vi "Periodic Tasks.vi"(8 "error in":errorcluster) -> ()   [LabVIEW 2016]
doc: "This VI runs in parallel to other tasks. It can contain as many user-defined periodic loops as you need. These can carry out PID or other sorts of timed response."
uses:
  <vilib>/Rock Robotics/WPI/Encoder/WPI_EncoderType.ctl
  <vilib>/Rock Robotics/SystemInterfaces/DIO/FPGA_DIOChannel.ctl
  <vilib>/Rock Robotics/WPI/Counter/WPI_CounterDigitalInputToDigitalSource.vi
  Encoder Rate Shooter.vi
  Shooter Distance.vi
  Encoder Distance.vi
  <vilib>/Rock Robotics/WPI/Utilities/WPI_GetSetVariantRefNum.vi
  Cam X.vi
  Cam Y.vi
  Cam H.vi
  Cam W.vi
  Ultrasonic distance.vi
  <vilib>/Rock Robotics/WPI/Ultrasonic/WPI_SonarSRF04DigitalClose.vi
  <vilib>/Rock Robotics/WPI/Ultrasonic/WPI_SonarSRF04DigitalOpen.vi
  <vilib>/Rock Robotics/WPI/Ultrasonic/WPI_SonarSRF04DigitalGetRange.vi
panel:
  out "Height":dbl
  out "Width":dbl
  out "Y":dbl
  out "X":dbl
  in  "Average Bits":u8=3 max=15
  in  "Scaling factor (V/in)":dbl=0.0098
  in  "stop 3":bool
  out "distance":dbl(slide)=125.0 scale=0.0..250.0 scale format="%3d"
  out "Encoder Direction 2":string
  out "Encoder Alarm Status 2":string
  in  "Reset Encoder? 2":bool
  in  "stop 2":bool
  out "Encoder Distance 2":dbl
  out "Encoder Rate (distance/sec) 2":dbl
  in  "Minimum Rate 2":dbl=20.0
  in  "A Channel 2":T1=enum."DIO 2"
  in  "B Channel 2":T1=enum."DIO 3"
  in  "DistancePerCount 2":dbl=1.0
  in  "Decoding Type 2":T2=enum."4x"
  in  "Invert Direction 2":bool=TRUE
  in  "Number Samples to Average 2":u8=4 min=1 max=128
  out "Encoder Direction":string
  out "Encoder Alarm Status":string
  in  "Reset Encoder?":bool
  in  "stop":bool
  out "Encoder Distance":dbl
  out "Encoder Rate (distance/sec)":dbl
  in  "Minimum Rate":dbl=20.0
  in  "A Channel":T1
  in  "B Channel":T1=enum."DIO 1"
  in  "DistancePerCount":dbl=1.0
  in  "Decoding Type":T2=enum."4x"
  in  "Invert Direction":bool
  in  "Number Samples to Average":u8=4 min=1 max=128
  # "DO NOT INVERT"
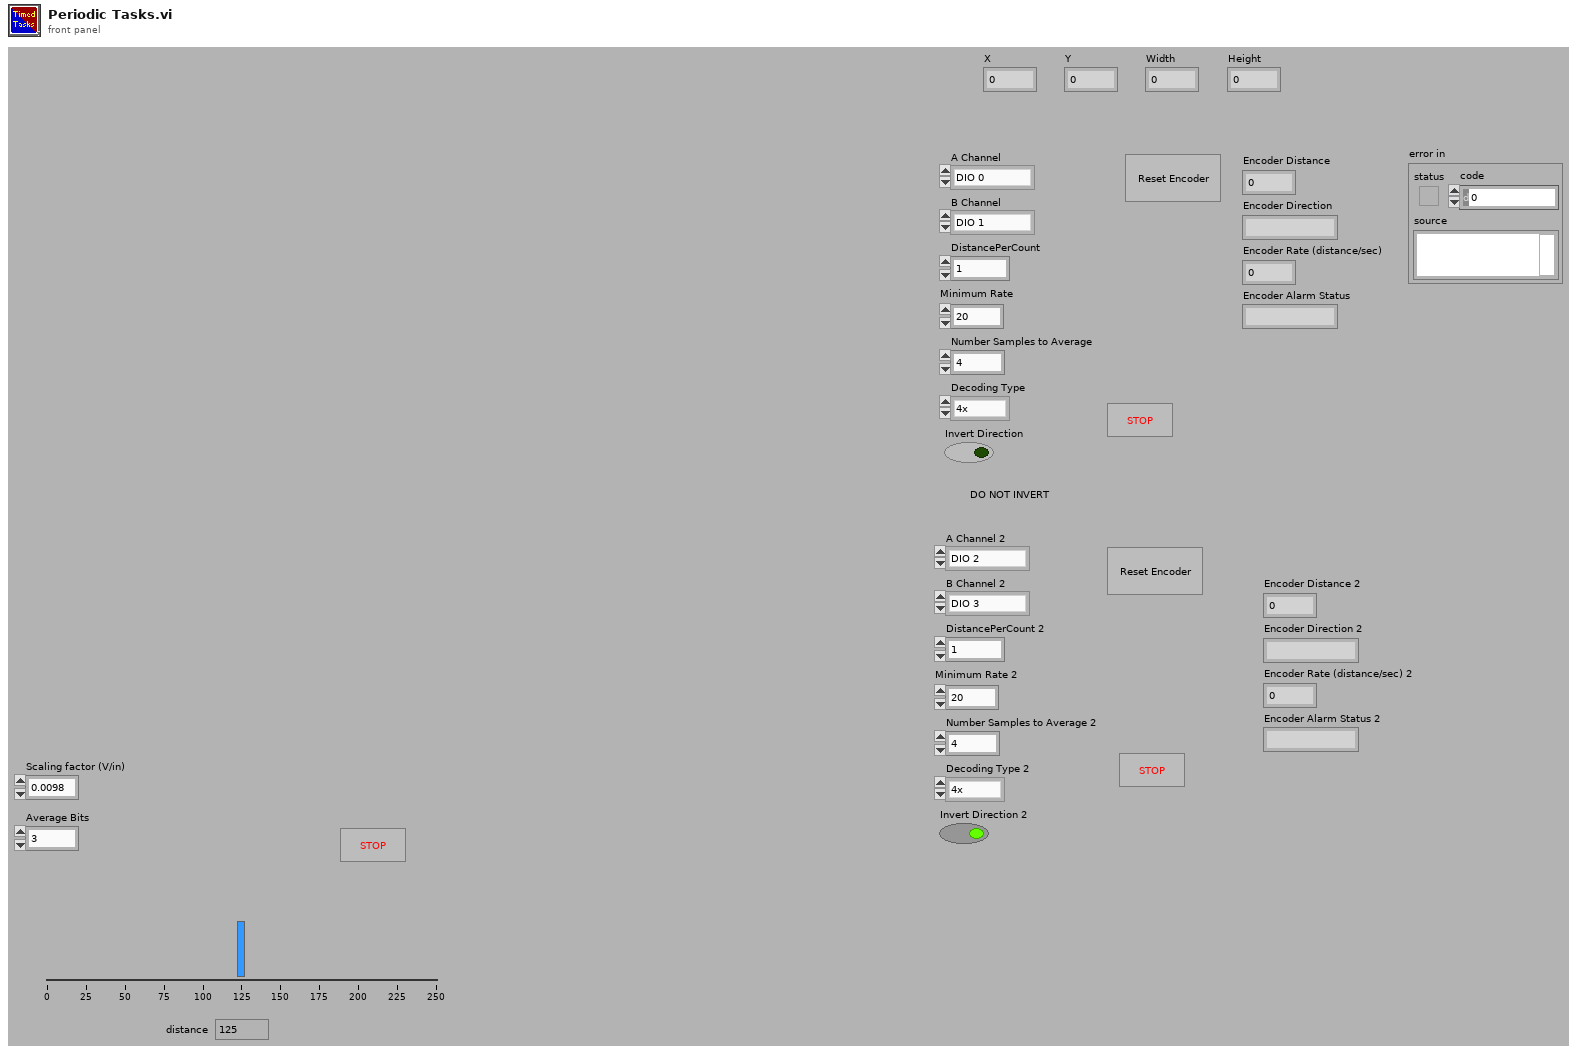
[diagram p1: front panel]
types:
  T1 = typedef "FPGA_DIOChannel.ctl" = enum8{"DIO 0", "DIO 1", "DIO 2", "DIO 3", "DIO 4", "DIO 5", "DIO 6", "DIO 7", "DIO 8", "DIO 9", "DIO MXP 0", "DIO MXP 1", "DIO MXP 2", "DIO MXP 3", "DIO MXP 4", "DIO MXP 5", "DIO MXP 6", "DIO MXP 7", "DIO MXP 8", "DIO MXP 9", "DIO MXP 10", "DIO MXP 11", "DIO MXP 12", "DIO MXP 13", "DIO MXP 14", "DIO MXP 15", "SPI Port CS1", "SPI Port CS2", "SPI Port CS3", "SPI Port MISO", "SPI Port MOSI", "Invalid"}
  T2 = typedef "WPI_EncoderType.ctl" = enum16{"1x", "2x", "4x"}
  T3 = typedef "WPI_DigitalInputDevRef.ctl" = cluster{"DevStatus":errorcluster, "DIO Channel":T1}
  T4 = typedef "FPGA_CounterEncoderSourceConvertionLVSourceType.ctl" = cluster{"DevStatus":errorcluster, "AnalogTriggerMode?":bool, "DigitalMode":cluster{"DIO Channel":T5}, "AnalogTriggerMode":cluster{"AnalogTriggerIndex":T6, "OutputType":T7}}
  T5 = typedef "FPGA_DIODigitalSourceChannel.ctl" = enum8{"DIO 0", "DIO 1", "DIO 2", "DIO 3", "DIO 4", "DIO 5", "DIO 6", "DIO 7", "DIO 8", "DIO 9", "DIO MXP 0", "DIO MXP 1", "DIO MXP 2", "DIO MXP 3", "DIO MXP 4", "DIO MXP 5", "DIO MXP 6", "DIO MXP 7", "DIO MXP 8", "DIO MXP 9", "DIO MXP 10", "DIO MXP 11", "DIO MXP 12", "DIO MXP 13", "DIO MXP 14", "DIO MXP 15", "Disabled"}
  T6 = typedef "FPGA_AnalogTriggerIndex.ctl" = enum8{"Trig 0", "Trig 1", "Trig 2", "Trig 3", "Trig 4", "Trig 5", "Trig 6", "Trig 7", "Invalid"}
  T7 = typedef "FPGA_AnalogTriggerOutType.ctl" = enum16{"InWindow", "TriggerState", "Rising", "Falling"}
  T8 = typedef "WPI_UltrasonicDeviceRef.ctl" = cluster{"DevStatus":errorcluster, "Ping Channel":T1, "Echo Channel":T1, "CntIndex":T9}
  T9 = typedef "FPGA_CounterCtrSystemIndex.ctl" = enum8{"Ctr 0", "Ctr 1", "Ctr 2", "Ctr 3", "Ctr 4", "Ctr 5", "Ctr 6", "Ctr 7", "Invalid"}
  T10 = typedef "WPI_EncoderDevRef.ctl" = cluster{"DevStatus":errorcluster, "EncoderIndex":T11, "CounterIndex":T9, "DistancePerCount":dbl, "Decoding Type":T2}
  T11 = typedef "FPGA_EncoderIdx.ctl" = enum8{"Enc 0", "Enc 1", "Enc 2", "Enc 3", "Enc 4", "Enc 5", "Enc 6", "Enc 7", "Invalid"}
  T12 = typedef "WPI_JoystickDevRef.ctl" = cluster{"Device":T13}
  T13 = typedef "WPI_JoystickDeviceEnum.ctl" = enum16{"USB 0", "USB 1", "USB 2", "USB 3", "USB 4", "USB 5"}
  T14 = typedef "WPI_RobotDriveDevRef.ctl" = cluster{"DevStatus":errorcluster, "Motors[]":T15[], "Square Inputs":bool, "Max Output":dbl}
  T15 = typedef "WPI_MotorControlDeviceRef.ctl" = cluster{"DeviceStatus":errorcluster, "Type":T16, "PWM":cluster{"PWM Channel":T17, "DeadBand":T18}, "CAN":cluster{"Device Number":u8, "SetOutput VI Ref":variant, "GetOutput VI Ref":variant, "Enable VI Ref":variant, "Disable VI Ref":variant, "Data":variant}, "Invert":bool}
  T16 = typedef "WPI_MotorControlType.ctl" = enum16{"PWM", "CAN"}
  T17 = typedef "FPGA_DIOPWMChannel.ctl" = enum8{"PWM 0", "PWM 1", "PWM 2", "PWM 3", "PWM 4", "PWM 5", "PWM 6", "PWM 7", "PWM 8", "PWM 9", "PWM MXP 0", "PWM MXP 1", "PWM MXP 2", "PWM MXP 3", "PWM MXP 4", "PWM MXP 5", "PWM MXP 6", "PWM MXP 7", "PWM MXP 8", "PWM MXP 9", "Invalid"}
  T18 = typedef "WPI_PWMDeadband.ctl" = cluster{"Name":string, "maxPositivePwm":i32, "minPositivePwm":i32, "centerPwm":i32, "maxNegativePwm":i32, "minNegativePwm":i32, "angularRange":u16}
  T19 = cluster{"JoystickDevRef":T12, "RobotDriveDevRef":T14}
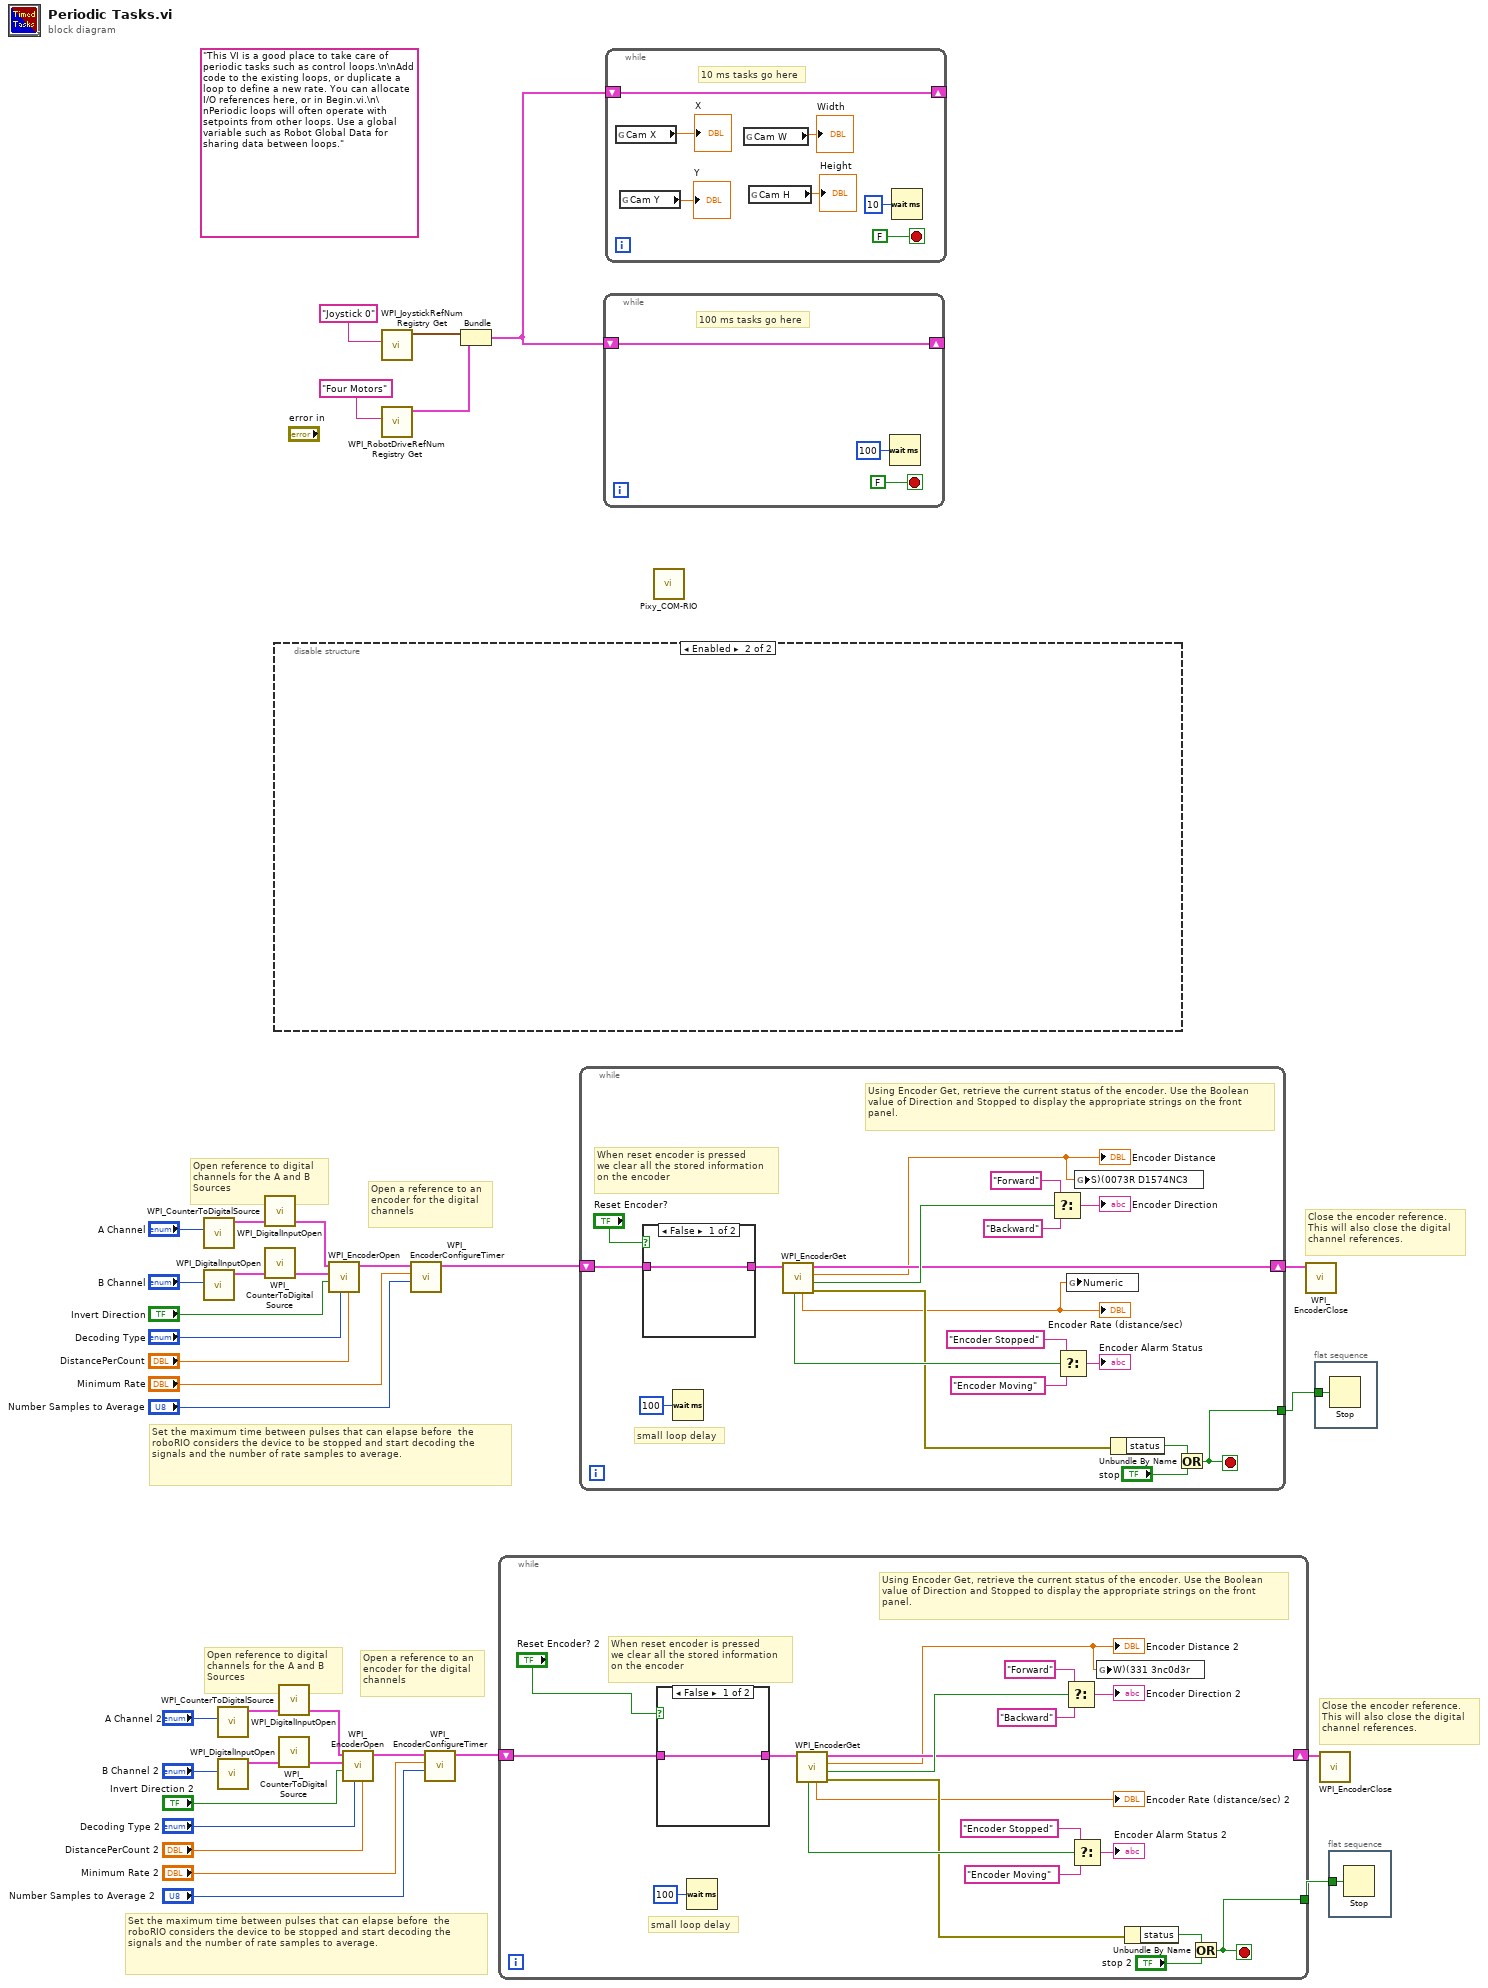
[diagram p0: block diagram]
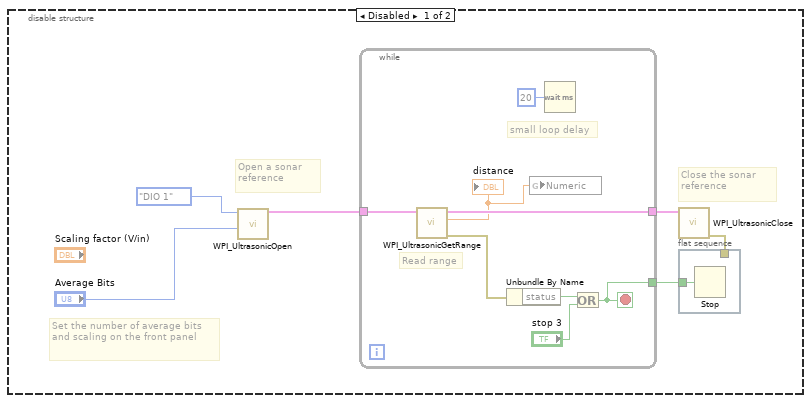
[diagram p2: hidden frame]
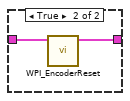
[diagram p3: hidden frame]
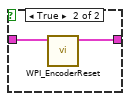
[diagram p4: hidden frame]
diagram:
  (unwired) "This VI is a good place to take care of periodic tasks such as control loops.\n\nAdd code to the existing loops, or duplicate a loop to define a new rate. You can allocate I/O references here, or in Begin.vi.\n\nPeriodic loops will often operate with setpoints from other loops. Use a global variable such as Robot Global Data for sharing data between loops."
  # "Close the encoder reference.\nThis will also close the digital \nchannel references."
  # "Set the maximum time between pulses that can elapse before  the roboRIO considers the device to be stopped and start decoding the signals and the number of rate samples to average."
  # "Open a reference to an\nencoder for the digital \nchannels"
  # "Open reference to digital \nchannels for the A and B\nSources"
  # "Close the encoder reference.\nThis will also close the digital \nchannel references."
  # "Set the maximum time between pulses that can elapse before  the roboRIO considers the device to be stopped and start decoding the signals and the number of rate samples to average."
  # "Open a reference to an\nencoder for the digital \nchannels"
  # "Open reference to digital \nchannels for the A and B\nSources"
  n1 = call <vilib>:"WPI_DigitalInputOpen.vi"("DIO Channel"="A Channel") -> ("DigitalInputDevRef"=w25:T3)  [unwired: 1 in, 9 out]
  n2 = call <vilib>:"WPI_DigitalInputOpen.vi"("DIO Channel"="B Channel") -> ("DigitalInputDevRef"=w24:T3)  [unwired: 1 in, 9 out]
  n3 = call <vilib>:"WPI_DigitalInputOpen.vi"("DIO Channel"="A Channel 2") -> ("DigitalInputDevRef"=w16:T3)  [unwired: 1 in, 9 out]
  n4 = call <vilib>:"WPI_DigitalInputOpen.vi"("DIO Channel"="B Channel 2") -> ("DigitalInputDevRef"=w17:T3)  [unwired: 1 in, 9 out]
  n5 = call-poly <vilib>:"WPI_CounterToDigitalSource.vi"("DigitalInputDevRef"=w25) -> ("Digital Source"=w26:T4)  [unwired: 6 out]
  n6 = call-poly <vilib>:"WPI_CounterToDigitalSource.vi"("DigitalInputDevRef"=w24) -> ("Digital Source"=w23:T4)  [unwired: 6 out]
  n7 = disable-structure shown="Enabled" {
    frame Disabled {
      # "Set the number of average bits and scaling on the front panel"
      # "Close the sonar reference"
      # "Open a sonar reference"
      n8 = call-poly <vilib>:"WPI_UltrasonicOpen.vi"("Echo DIO Channel"="Average Bits", "Ping DIO Channel"=FPGA_DIOChannel."DIO 1") -> ("SonarSRF04DevRef"=w40:T8)  [unwired: 8 in, 1 out]
      n9 = while {
        tunnel: w40 -> [w44]
        tunnel: [w50] -> w38
        tunnel: [w45] -> w41
        stop <- w45 stop-if-true
        # "small loop delay"
        # "Read range"
        n10 = call-poly <vilib>:"WPI_UltrasonicGetRange.vi"("SonarSRF04DevRef"=w44) -> ("error out"=w46:errorcluster, "Distance"=w43:dbl, "SonarSRF04DevRef"=w50:T8)  [unwired: 8 in]
        "distance" <- w43
        n11 = Unbundle By Name(w46) -> ("status"=w48:bool)
        n12 = global write "Ultrasonic distance.vi" "Numeric"(w43) -> ()
        n13 = Wait (ms)(milliseconds to wait=u32 20) -> ()  [unwired: 1 out]
        n14 = Or(x=w48, y="stop 3") -> (x .or. y?=w45:bool)
      }
      n15 = call-poly <vilib>:"WPI_UltrasonicClose.vi"("SonarSRF04DevRef"=w38) -> ("error out"=w37:errorcluster)  [unwired: 10 in]
      n16 = flat-sequence {
        tunnel: w41 -> [w42]
        tunnel: w37 -> [_]
        frame #0 {
          n17 = Stop(stop? (T)=w42) -> ()
        }
      }
    }
    frame Enabled {
    }
  }
  n18 = call-poly <vilib>:"WPI_CounterToDigitalSource.vi"("DigitalInputDevRef"=w16) -> ("Digital Source"=w15:T4)  [unwired: 6 out]
  n19 = call-poly <vilib>:"WPI_CounterToDigitalSource.vi"("DigitalInputDevRef"=w17) -> ("Digital Source"=w18:T4)  [unwired: 6 out]
  n20 = call <vilib>:"WPI_EncoderOpen.vi"("DistancePerCount"="DistancePerCount", "Decoding Type"="Decoding Type", "Invert Direction (False)"="Invert Direction", "BSource"=w23, "ASource"=w26) -> ("EncoderDevRef"=w33:T10)  [unwired: 3 in, 3 out]
  n21 = call <vilib>:"WPI_EncoderOpen.vi"("DistancePerCount"="DistancePerCount 2", "Decoding Type"="Decoding Type 2", "Invert Direction (False)"="Invert Direction 2", "BSource"=w18, "ASource"=w15) -> ("EncoderDevRef"=w8:T10)  [unwired: 3 in, 3 out]
  n22 = call <vilib>:"WPI_JoystickRefNum Registry Get.vi"("refnum name"="Joystick 0") -> ("JoystickDevRef"=w3:T12)  [unwired: 1 in, 9 out]
  n23 = call <vilib>:"WPI_RobotDriveRefNum Registry Get.vi"("refnum name"="Four Motors") -> ("RobotDriveDevRef"=w2:T14)  [unwired: 1 in, 9 out]
  n24 = call <vilib>:"WPI_EncoderConfigureTimer.vi"("Number Samples to Average"="Number Samples to Average", "Minimum Rate"="Minimum Rate", "EncoderDevRef"=w33) -> ("EncoderDevRef"=w32:T10)  [unwired: 1 in, 7 out]
  n25 = call <vilib>:"WPI_EncoderConfigureTimer.vi"("Number Samples to Average"="Number Samples to Average 2", "Minimum Rate"="Minimum Rate 2", "EncoderDevRef"=w8) -> ("EncoderDevRef"=w9:T10)  [unwired: 1 in, 7 out]
  n26 = Bundle("JoystickDevRef"=w3, "RobotDriveDevRef"=w2) -> (w1:T19)  [unwired: 1 out]
  n27 = while {
    shift-right: [w64] -> w19
    shift-left: w9 -> [w69]
    tunnel: [w63] -> w20
    stop <- w63 stop-if-true
    # "small loop delay"
    # "Using Encoder Get, retrieve the current status of the encoder. Use the Boolean value of Direction and Stopped to display the appropriate strings on the front panel."
    # "When reset encoder is pressed\nwe clear all the stored information\non the encoder"
    n28 = case shown="False" "Reset Encoder? 2" {
      tunnel: w69 -> [w70 w72]
      tunnel: [w70 w71] -> w67
      frame False {
      }
      frame True {
        n29 = call <vilib>:"WPI_EncoderReset.vi"("EncoderDevRef"=w72) -> ("EncoderDevRef"=w71:T10)  [unwired: 1 in, 9 out]
      }
    }
    n30 = Wait (ms)(milliseconds to wait=u32 100) -> ()  [unwired: 1 out]
    n31 = call <vilib>:"WPI_EncoderGet.vi"("EncoderDevRef"=w67) -> ("error out"=w62:errorcluster, "Direction"=w66:bool, "Distance"=w52:dbl, "EncoderDevRef"=w64:T10, "Rate"=→"Encoder Rate (distance/sec) 2":dbl, "Stopped"=w65:bool)  [unwired: 1 in, 4 out]
    "Encoder Distance 2" <- w52
    n32 = Select(t="Forward", s=w66, f="Backward") -> (s? t:f=→"Encoder Direction 2":string)
    n33 = Select(t="Encoder Stopped", s=w65, f="Encoder Moving") -> (s? t:f=→"Encoder Alarm Status 2":string)
    n34 = global write "Encoder Distance.vi" "W)(331 3nc0d3r"(w52) -> ()
    n35 = Unbundle By Name(w62) -> ("status"=w60:bool)
    n36 = Or(x=w60, y="stop 2") -> (x .or. y?=w63:bool)
  }
  n37 = while {
    shift-right: [w86] -> w22
    shift-left: w32 -> [w91]
    tunnel: [w85] -> w21
    stop <- w85 stop-if-true
    # "small loop delay"
    # "Using Encoder Get, retrieve the current status of the encoder. Use the Boolean value of Direction and Stopped to display the appropriate strings on the front panel."
    # "When reset encoder is pressed\nwe clear all the stored information\non the encoder"
    n38 = case shown="False" "Reset Encoder?" {
      tunnel: w91 -> [w92 w94]
      tunnel: [w92 w93] -> w89
      frame False {
      }
      frame True {
        n39 = call <vilib>:"WPI_EncoderReset.vi"("EncoderDevRef"=w94) -> ("EncoderDevRef"=w93:T10)  [unwired: 1 in, 9 out]
      }
    }
    n40 = Wait (ms)(milliseconds to wait=u32 100) -> ()  [unwired: 1 out]
    n41 = call <vilib>:"WPI_EncoderGet.vi"("EncoderDevRef"=w89) -> ("error out"=w83:errorcluster, "Direction"=w88:bool, "Distance"=w73:dbl, "EncoderDevRef"=w86:T10, "Rate"=w74:dbl, "Stopped"=w87:bool)  [unwired: 1 in, 4 out]
    "Encoder Distance" <- w73
    "Encoder Rate (distance/sec)" <- w74
    n42 = Select(t="Forward", s=w88, f="Backward") -> (s? t:f=→"Encoder Direction":string)
    n43 = Select(t="Encoder Stopped", s=w87, f="Encoder Moving") -> (s? t:f=→"Encoder Alarm Status":string)
    n44 = global write "Encoder Rate Shooter.vi" "Numeric"(w74) -> ()
    n45 = global write "Shooter Distance.vi" "S)(0073R D1574NC3"(w73) -> ()
    n46 = Unbundle By Name(w83) -> ("status"=w81:bool)
    n47 = Or(x=w81, y="stop") -> (x .or. y?=w85:bool)
  }
  n48 = while {
    shift-right: [w95] -> _
    shift-left: w1 -> [w95]
    stop <- FALSE stop-if-true
    # "100 ms tasks go here"
    n49 = Wait (ms)(milliseconds to wait=u32 100) -> ()  [unwired: 1 out]
  }
  n50 = while {
    shift-right: [w102] -> _
    shift-left: w1 -> [w102]
    stop <- FALSE stop-if-true
    # "10 ms tasks go here"
    n51 = global read "Cam X.vi" "Cam X"() -> (→"X":dbl)
    n52 = global read "Cam Y.vi" "Cam Y"() -> (→"Y":dbl)
    n53 = global read "Cam W.vi" "Cam W"() -> (→"Width":dbl)
    n54 = global read "Cam H.vi" "Cam H"() -> (→"Height":dbl)
    n55 = Wait (ms)(milliseconds to wait=u32 10) -> ()  [unwired: 1 out]
  }
  n56 = call "Pixy_COM-RIO.vi"() -> ()  [unwired: 7 in, 5 out]
  n57 = call <vilib>:"WPI_EncoderClose.vi"("EncoderDevRef"=w22) -> ()  [unwired: 2 in, 9 out]
  n58 = flat-sequence {
    tunnel: w21 -> [w105]
    frame #0 {
      n59 = Stop(stop? (T)=w105) -> ()
    }
  }
  n60 = call <vilib>:"WPI_EncoderClose.vi"("EncoderDevRef"=w19) -> ()  [unwired: 2 in, 9 out]
  n61 = flat-sequence {
    tunnel: w20 -> [w106]
    frame #0 {
      n62 = Stop(stop? (T)=w106) -> ()
    }
  }
